vi "Send Results Object.vi"(8 "error in (no error)":errorcluster, 10 "Results.lvclass":refnum<class "Results.lvclass">, 11 "Message Enqueuer in":refnum<class "Message Enqueuer.lvclass">) -> (0 "error out":errorcluster, 3 "Message Enqueuer out":refnum<class "Message Enqueuer.lvclass">)   [LabVIEW 2016, in "Controller Actor.lvlib" / "Send Results Object.lvclass"]
uses:
  <userlib>/Common Components/Controller/Messages/Send Results Object/Send Results Object.lvclass
  <userlib>/Common Components/Results/Results.lvclass
  <vilib>/ActorFramework/Message Enqueuer/Message Enqueuer.lvclass
  C:/Program Files (x86)/National Instruments/LabVIEW 2016/vi.lib/ActorFramework/Message/Message.lvclass
  <vilib>/ActorFramework/Message Enqueuer/Message Enqueuer.lvclass/Message Enqueuer.ctl
  <vilib>/ActorFramework/Message Priority Queue/Priority Enqueue.vi
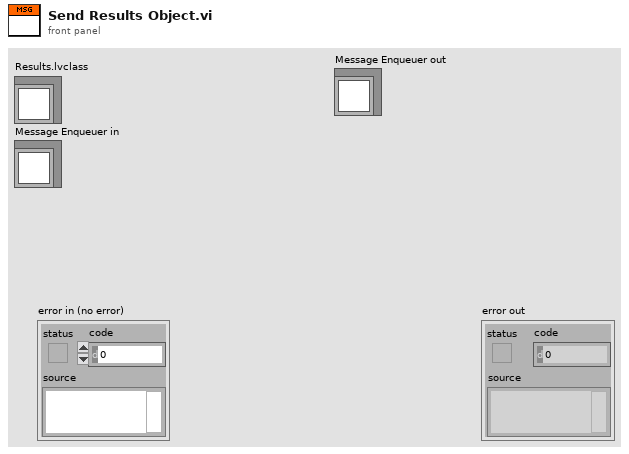
[diagram p1: front panel]
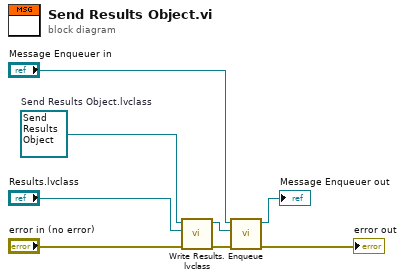
[diagram p0: block diagram]
diagram:
  w8 = refnum<class "Send Results Object.lvclass"> refnum  # Send Results Object.lvclass
  n1 = call <userlib>:"Write Results.lvclass.vi"("error in (no error)"="error in (no error)", "Results.lvclass"="Results.lvclass", "Send Results Object in"=w8) -> ("error out"=w5:errorcluster, "Send Results Object out"=w6:refnum<class "Send Results Object.lvclass">)  [unwired: 7 in]
  n2 = call <vilib>:"Enqueue.vi"("error in (no error)"=w5, "Message"=w6, "Message Enqueuer in"="Message Enqueuer in") -> ("error out"=→"error out":errorcluster, "Message Enqueuer out"=→"Message Enqueuer out":refnum<class "Message Enqueuer.lvclass">)  [unwired: 7 in]
